vi "UIProcessManipJoysticks.vi"(8 "Axes":dbl[](array[numeric]), 9 "POVs":i16[](array[numeric]), 10 "Buttons":bool[](array[boolean])) -> ()   [LabVIEW 2014, in "UILib.lvlib"]
uses:
  UILib.lvlib
  <vilib>/Rock Robotics/WPI/Solenoid/WPI_SolenoidValue.ctl
  LiftLib/LiftLib.lvlib
  LatchLib/LatchLib.lvlib
  GateLib/GateLib.lvlib
  IntakeLib/IntakeLib.lvlib
panel:
  in  "LatchLinkState":bool
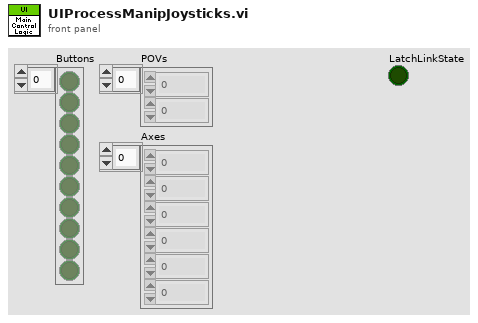
[diagram p1: front panel]
types:
  T1 = cluster{"Buttons[0]":bool, "Buttons[1]":bool, "Buttons[2]":bool, "Buttons[3]":bool, "Buttons[4]":bool, "Buttons[5]":bool, "Buttons[6]":bool, "Buttons[7]":bool, "Buttons[8]":bool}
  T2 = typedef "WPI_SolenoidValue.ctl" = enum16{"Off", "On", "Forward", "Reverse"}
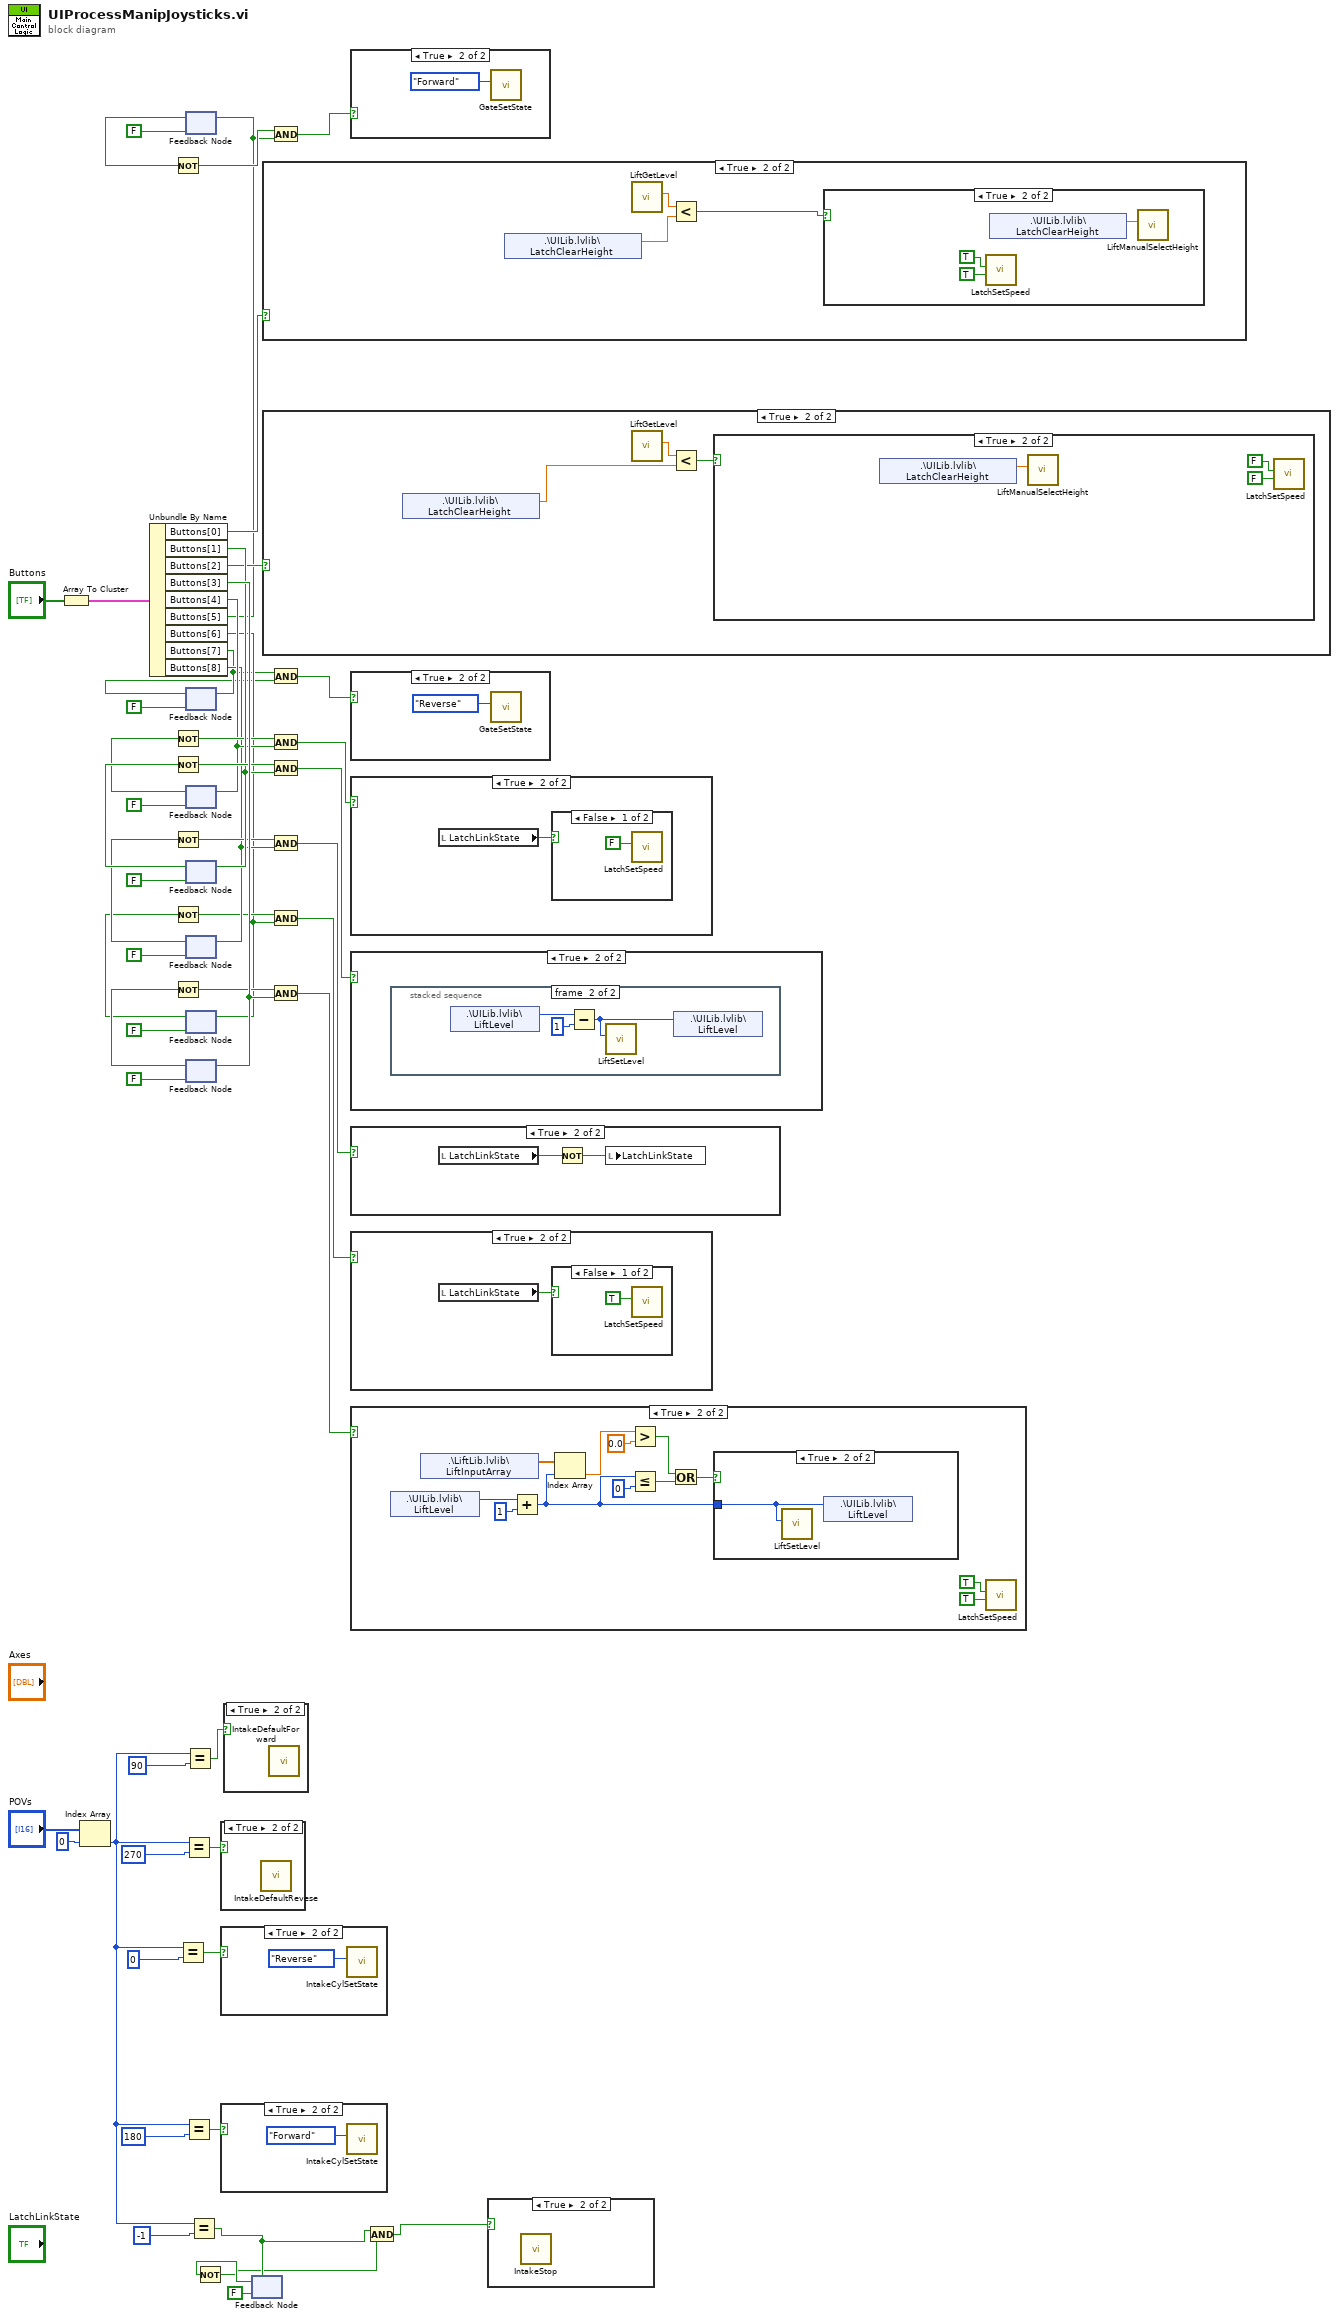
[diagram p0: block diagram]
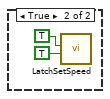
[diagram p10: hidden frame]
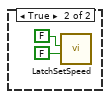
[diagram p13: hidden frame]
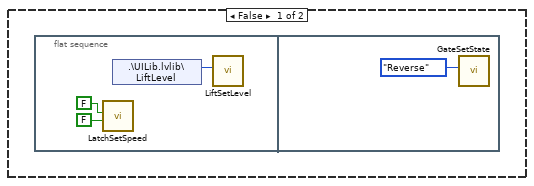
[diagram p15: hidden frame]
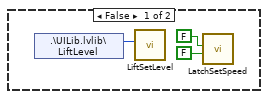
[diagram p17: hidden frame]
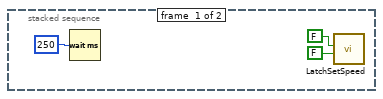
[diagram p19: hidden frame]
diagram:
  n1 = Array To Cluster(array="Buttons") -> (cluster=w54:T1)
  n2 = Index Array(array="POVs", index=0) -> (element=w6:i16)
  n3 = Unbundle By Name(w54) -> ("Buttons[0]"=w28:bool, "Buttons[1]"=w44:bool, "Buttons[2]"=w43:bool, "Buttons[3]"=w52:bool, "Buttons[4]"=w34:bool, "Buttons[5]"=w23:bool, "Buttons[6]"=w27:bool, "Buttons[7]"=w20:bool, "Buttons[8]"=w33:bool)
  n4 = Equal?(x=w6, y=i16 0) -> (x = y?=w12:bool)
  n5 = Equal?(x=w6, y=i16 270) -> (x = y?=w14:bool)
  n6 = Equal?(x=w6, y=i16 180) -> (x = y?=w11:bool)
  n7 = Equal?(x=w6, y=i16 90) -> (x = y?=w8:bool)
  n8 = feedback #1(FALSE ("Buttons[3]")) -> (w25:bool)
  n9 = Not(x=w25) -> (.not. x?=w24:bool)
  n10 = feedback-in #1(w23) -> ()
  n11 = feedback #2(FALSE ("Buttons[3]")) -> (w19:bool)
  n12 = feedback-in #2(w20) -> ()
  n13 = feedback #3(FALSE ("Buttons[3]")) -> (w42:bool)
  n14 = Not(x=w42) -> (.not. x?=w40:bool)
  n15 = feedback-in #3(w34) -> ()
  n16 = feedback #4(FALSE ("Buttons[3]")) -> (w47:bool)
  n17 = Not(x=w47) -> (.not. x?=w46:bool)
  n18 = feedback-in #4(w44) -> ()
  n19 = feedback #5(FALSE ("Buttons[3]")) -> (w37:bool)
  n20 = Not(x=w37) -> (.not. x?=w36:bool)
  n21 = feedback-in #5(w33) -> ()
  n22 = feedback #6(FALSE ("Buttons[5]")) -> (w31:bool)
  n23 = Not(x=w31) -> (.not. x?=w30:bool)
  n24 = feedback-in #6(w27) -> ()
  n25 = feedback-in #7(w52) -> ()
  n26 = feedback #7(FALSE ("Buttons[3]")) -> (w51:bool)
  n27 = Not(x=w51) -> (.not. x?=w50:bool)
  n28 = Equal?(x=w6, y=i16 -1) -> (x = y?=w3:bool)
  n29 = case shown="True" w14 {
    frame False {
    }
    frame True {
      n30 = call "IntakeDefaultRevese.vi"() -> ()  [unwired: 12 in]
    }
  }
  n31 = case shown="True" w12 {
    frame False {
    }
    frame True {
      n32 = call "IntakeCylSetState.vi"("IntakeCylState"=WPI_SolenoidValue."Reverse") -> ()  [unwired: 11 in]
    }
  }
  n33 = case shown="True" w11 {
    frame False {
    }
    frame True {
      n34 = call "IntakeCylSetState.vi"("IntakeCylState"=WPI_SolenoidValue."Forward") -> ()  [unwired: 11 in]
    }
  }
  n35 = case shown="True" w8 {
    frame False {
    }
    frame True {
      n36 = call "IntakeDefaultForward.vi"() -> ()  [unwired: 12 in]
    }
  }
  n37 = feedback-in #8(w3) -> ()
  n38 = feedback #8(FALSE) -> (w4:bool)
  n39 = Not(x=w4) -> (.not. x?=w2:bool)
  n40 = case shown="True" w28 {
    frame False {
    }
    frame True {
      n41 = shared-variable ".\\UILib.lvlib\\LatchClearHeight"() -> (w58:dbl)  [unwired: 1 in, 1 out]
      n42 = call "LiftGetLevel.vi"() -> ("LiftCurrentHeight"=w60:dbl)  [unwired: 11 in]
      n43 = Less?(x=w60, y=w58) -> (x < y?=w59:bool)
      n44 = case shown="True" w59 {
        frame False {
          n45 = shared-variable ".\\UILib.lvlib\\LiftLevel"() -> (w61:i32)  [unwired: 1 in, 1 out]
          n46 = call "LiftSetLevel.vi"("Index"=w61) -> ()  [unwired: 11 in]
          n47 = call "LatchSetSpeed.vi"("LatchContainerState"=FALSE, "LatchLatchState"=FALSE) -> ()  [unwired: 10 in]
        }
        frame True {
          n48 = call "LatchSetSpeed.vi"("LatchContainerState"=TRUE, "LatchLatchState"=TRUE) -> ()  [unwired: 10 in]
          n49 = shared-variable ".\\UILib.lvlib\\LatchClearHeight"() -> (w66:dbl)  [unwired: 1 in, 1 out]
          n50 = call "LiftManualSelectHeight.vi"("Height"=w66) -> ()  [unwired: 11 in]
        }
      }
    }
  }
  n51 = case shown="True" w43 {
    frame False {
    }
    frame True {
      n52 = shared-variable ".\\UILib.lvlib\\LatchClearHeight"() -> (w67:dbl)  [unwired: 1 in, 1 out]
      n53 = call "LiftGetLevel.vi"() -> ("LiftCurrentHeight"=w69:dbl)  [unwired: 11 in]
      n54 = Less?(x=w69, y=w67) -> (x < y?=w68:bool)
      n55 = case shown="True" w68 {
        frame False {
          n56 = flat-sequence {
            frame #0 {
              n57 = call "LatchSetSpeed.vi"("LatchContainerState"=FALSE, "LatchLatchState"=FALSE) -> ()  [unwired: 10 in]
              n58 = shared-variable ".\\UILib.lvlib\\LiftLevel"() -> (w72:i32)  [unwired: 1 in, 1 out]
              n59 = call "LiftSetLevel.vi"("Index"=w72) -> ()  [unwired: 11 in]
            }
            frame #1 {
              n60 = call "GateSetState.vi"("GateCylState"=WPI_SolenoidValue."Reverse") -> ()  [unwired: 11 in]
            }
          }
        }
        frame True {
          n61 = shared-variable ".\\UILib.lvlib\\LatchClearHeight"() -> (w76:dbl)  [unwired: 1 in, 1 out]
          n62 = call "LiftManualSelectHeight.vi"("Height"=w76) -> ()  [unwired: 11 in]
          n63 = call "LatchSetSpeed.vi"("LatchContainerState"=FALSE, "LatchLatchState"=FALSE) -> ()  [unwired: 10 in]
        }
      }
    }
  }
  n64 = And(x=w24, y=w23) -> (x .and. y?=w22:bool)
  n65 = And(x=w20, y=w19) -> (x .and. y?=w18:bool)
  n66 = And(x=w40, y=w34) -> (x .and. y?=w39:bool)
  n67 = And(x=w46, y=w44) -> (x .and. y?=w45:bool)
  n68 = And(x=w36, y=w33) -> (x .and. y?=w35:bool)
  n69 = And(x=w30, y=w27) -> (x .and. y?=w29:bool)
  n70 = And(x=w50, y=w52) -> (x .and. y?=w49:bool)
  n71 = case shown="True" w22 {
    frame False {
    }
    frame True {
      n72 = call "GateSetState.vi"("GateCylState"=WPI_SolenoidValue."Forward") -> ()  [unwired: 11 in]
    }
  }
  n73 = case shown="True" w18 {
    frame False {
    }
    frame True {
      n74 = call "GateSetState.vi"("GateCylState"=WPI_SolenoidValue."Reverse") -> ()  [unwired: 11 in]
    }
  }
  n75 = case shown="True" w39 {
    frame False {
    }
    frame True {
      n76 = local read "LatchLinkState"() -> (w79:bool)
      n77 = case shown="False" w79 {
        frame False {
          n78 = call "LatchSetSpeed.vi"("LatchLatchState"=FALSE) -> ()  [unwired: 11 in]
        }
        frame True {
          n79 = call "LatchSetSpeed.vi"("LatchContainerState"=FALSE, "LatchLatchState"=FALSE) -> ()  [unwired: 10 in]
        }
      }
    }
  }
  n80 = case shown="True" w45 {
    frame False {
    }
    frame True {
      n81 = stacked-sequence {
        frame #0 {
          n82 = Wait (ms)(milliseconds to wait=u32 250) -> ()  [unwired: 1 out]
          n83 = call "LatchSetSpeed.vi"("LatchContainerState"=FALSE, "LatchLatchState"=FALSE) -> ()  [unwired: 10 in]
        }
        frame #1 {
          n84 = shared-variable ".\\UILib.lvlib\\LiftLevel"() -> (w86:i32)  [unwired: 1 in, 1 out]
          n85 = Subtract(x=w86, y=1) -> (x-y=w87:i32)
          n86 = call "LiftSetLevel.vi"("Index"=w87) -> ()  [unwired: 11 in]
          n87 = shared-variable ".\\UILib.lvlib\\LiftLevel"(w87) -> ()  [unwired: 1 in, 1 out]
        }
      }
    }
  }
  n88 = case shown="True" w35 {
    frame False {
    }
    frame True {
      n89 = local read "LatchLinkState"() -> (w90:bool)
      n90 = Not(x=w90) -> (.not. x?=w89:bool)
      n91 = local write "LatchLinkState"(w89) -> ()
    }
  }
  n92 = case shown="True" w29 {
    frame False {
    }
    frame True {
      n93 = local read "LatchLinkState"() -> (w91:bool)
      n94 = case shown="False" w91 {
        frame False {
          n95 = call "LatchSetSpeed.vi"("LatchLatchState"=TRUE) -> ()  [unwired: 11 in]
        }
        frame True {
          n96 = call "LatchSetSpeed.vi"("LatchContainerState"=TRUE, "LatchLatchState"=TRUE) -> ()  [unwired: 10 in]
        }
      }
    }
  }
  n97 = case shown="True" w49 {
    frame False {
    }
    frame True {
      n98 = shared-variable ".\\UILib.lvlib\\LiftLevel"() -> (w106:i32)  [unwired: 1 in, 1 out]
      n99 = shared-variable ".\\LiftLib.lvlib\\LiftInputArray"() -> (w102:dbl[])  [unwired: 1 in, 1 out]
      n100 = Add(x=w106, y=1) -> (x+y=w98:i32)
      n101 = Index Array(array=w102, index=w98) -> (element=w101:dbl)
      n102 = Greater?(x=w101, y=0.0) -> (0:w99:bool)
      n103 = Less Or Equal?(x=w98, y=0) -> (x <= y?=w96:bool)
      n104 = Or(x=w99, y=w96) -> (x .or. y?=w95:bool)
      n105 = case shown="True" w95 {
        tunnel: w98 -> [_ w107]
        frame False {
        }
        frame True {
          n106 = call "LiftSetLevel.vi"("Index"=w107) -> ()  [unwired: 11 in]
          n107 = shared-variable ".\\UILib.lvlib\\LiftLevel"(w107) -> ()  [unwired: 1 in, 1 out]
        }
      }
      n108 = call "LatchSetSpeed.vi"("LatchContainerState"=TRUE, "LatchLatchState"=TRUE) -> ()  [unwired: 10 in]
    }
  }
  n109 = And(x=w3, y=w2) -> (x .and. y?=w1:bool)
  n110 = case shown="True" w1 {
    frame False {
    }
    frame True {
      n111 = call "IntakeStop.vi"() -> ()  [unwired: 12 in]
    }
  }
